vi "Read Requestor.vi"(8 "error in (no error)":errorcluster, 11 "Recieve Request for Result Msg in":refnum<class "Recieve Request for Result Msg.lvclass">) -> (0 "error out":errorcluster, 2 "Requestor":string, 3 "Recieve Request for Result Msg out":refnum<class "Recieve Request for Result Msg.lvclass">)   [LabVIEW 2015, in "Recieve Request for Result Msg.lvclass"]
uses:
  Recieve Request for Result Msg.lvclass
  Recieve Request for Result Msg.lvclass/Recieve Request for Result Msg.ctl
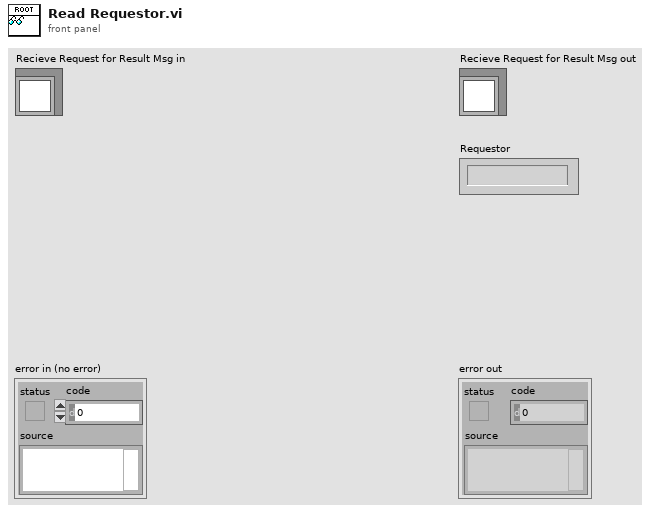
[diagram p1: front panel]
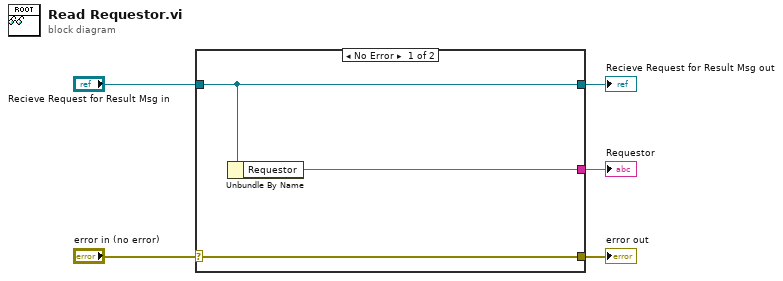
[diagram p0: block diagram]
diagram:
  n1 = case shown="No Error" "error in (no error)" {
    selector: "error in (no error)" -> [w8 w9]
    tunnel: [w8 w9] -> w4
    tunnel: [w7 w10] -> w2
    tunnel: "Recieve Request for Result Msg in" -> [w7 w10]
    tunnel: [w6 _] -> w1
    frame No Error {
      n2 = Unbundle By Name(w7) -> ("Requestor"=w6:string)
    }
    frame Error {
    }
  }
  "error out" <- w4
  "Recieve Request for Result Msg out" <- w2
  "Requestor" <- w1
